vi "GenericScpiRW.vi"(8 "error in (no error)":errorcluster, 9 "Query?":bool, 10 "SCPI Command":string, 11 "resource name":refnum<k15>) -> (0 "error out":errorcluster, 2 "SCPI Response":string)   [LabVIEW 2014]
doc: "Allows the user to send standard SCPI commands/queries."
uses:
  <instrlib>/Agilent NA/Agilent NA.lvlib
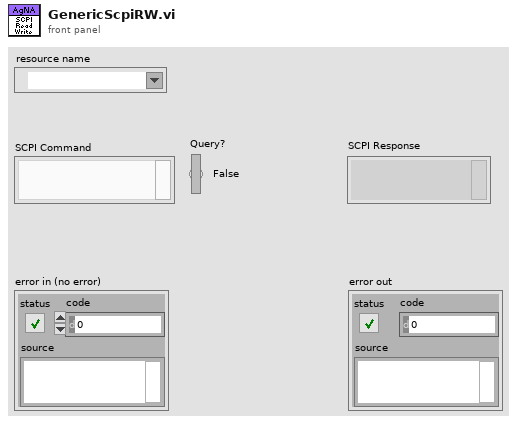
[diagram p1: front panel]
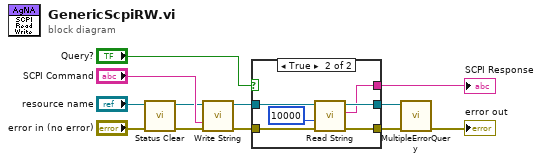
[diagram p0: block diagram]
diagram:
  n1 = call <instrlib>:"Status Clear.vi"("error in (no error)"="error in (no error)", "instrument handle"="resource name") -> ("error out"=w2:errorcluster, "instrument handle out"=w1:refnum<k15>)  [unwired: 8 in]
  n2 = call <instrlib>:"Write String.vi"("error in (no error)"=w2, "Command"="SCPI Command", "instrument handle"=w1) -> ("error out"=w8:errorcluster, "instrument handle out"=w9:refnum<k15>)  [unwired: 7 in]
  n3 = case shown="True" "Query?" {
    tunnel: w8 -> [w13 w20]
    tunnel: w9 -> [w14 w19]
    tunnel: [w13 w18] -> w10
    tunnel: [w14 w17] -> w12
    tunnel: [_ w16] -> w11
    frame False {
    }
    frame True {
      n4 = call <instrlib>:"Read String.vi"("error in (no error)"=w20, "ValBufferSize"=10000, "instrument handle"=w19) -> ("error out"=w18:errorcluster, "Val"=w16:string, "instrument handle out"=w17:refnum<k15>)  [unwired: 6 in]
    }
  }
  "SCPI Response" <- w11
  n5 = call "MultipleErrorQuery.vi"("error in (no error)"=w10, "instrument handle"=w12) -> ("error out"=→"error out":errorcluster)  [unwired: 7 in, 2 out]
